vi "Logger.PGSQL.Disconnect.vi"(8 "error in (no error)":errorcluster, 11 "Logger.PGSQL in":refnum<class "Logger.PGSQL.lvclass">) -> (0 "error out":errorcluster, 3 "Logger.PGSQL out":refnum<class "Logger.PGSQL.lvclass">)   [LabVIEW 2019, in "Logger.PGSQL.lvlib" / "Logger.PGSQL.lvclass"]
uses:
  Logger.PGSQL.lvclass
  Logger.PGSQL.lvclass/Logger.PGSQL.ctl
  <userlib>/LevyLab/LV-Data/LV-Data.PG/LV-Data.PGSQL.lvclass
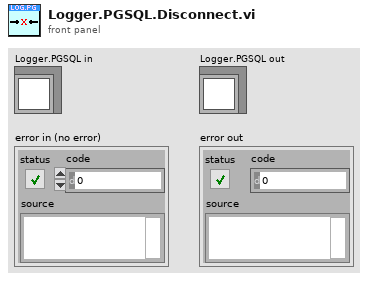
[diagram p1: front panel]
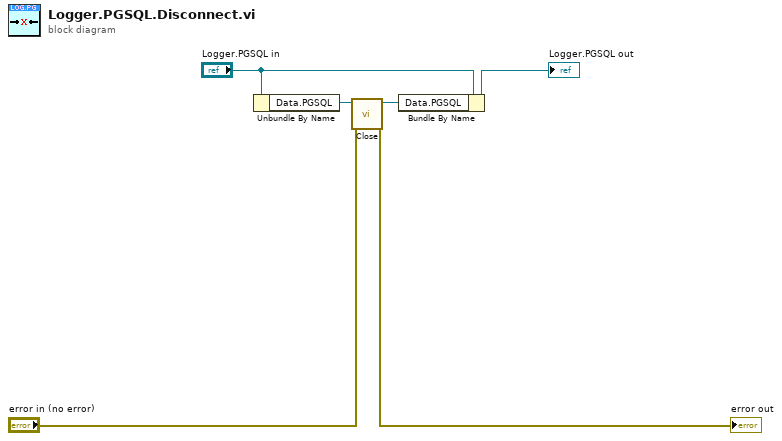
[diagram p0: block diagram]
diagram:
  n1 = Unbundle By Name("Logger.PGSQL in") -> ("Data.PGSQL"=w3:refnum<class "LV-Data.PGSQL.lvclass">)
  n2 = call-dynamic "Close.vi"("error in (no error)"="error in (no error)", "Data.PG in"=w3) -> ("error out"=→"error out":errorcluster, "Data.PG out"=w4:refnum<class "LV-Data.PGSQL.lvclass">)  [unwired: 8 in]
  n3 = Bundle By Name(cluster="Logger.PGSQL in", "Data.PGSQL"=w4) -> (→"Logger.PGSQL out":refnum<class "Logger.PGSQL.lvclass">)
